vi "Init Events.vi"(8 "error in (no error)":errorcluster, 11 "BluelinesRedlines in":refnum<class "BluelinesRedlines.lvclass">) -> (0 "error out":errorcluster, 3 "BluelinesRedlines out":refnum<class "BluelinesRedlines.lvclass">)   [LabVIEW 2020, in "VolatusGUIElements.lvlib" / "BluelinesRedlines.lvclass"]
uses:
  BluelinesRedlines.lvclass
  Value Change Data.ctl
  BLRL Control.ctl
  Events.ctl
  BluelinesRedlines.lvclass/BluelinesRedlines.ctl
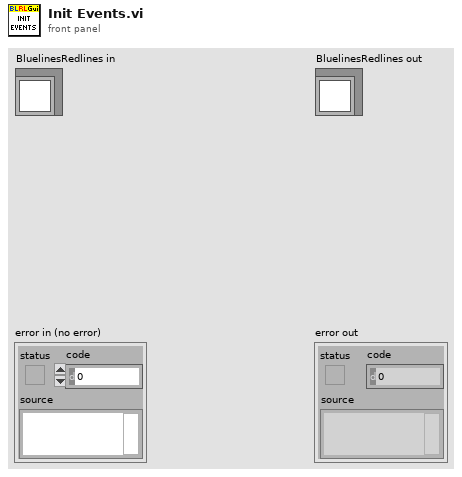
[diagram p1: front panel]
types:
  T1 = typedef "VolatusGUIElements.lvlib/BluelinesRedlines.lvclass/Events.ctl" = cluster{"Value Change":refnum<user-event>, "Disabled":refnum<user-event>}
  T2 = typedef "VolatusGUIElements.lvlib/BluelinesRedlines.lvclass/Value Change Data.ctl" = cluster{"Old":T3, "New":T3}
  T3 = typedef "VolatusGUIElements.lvlib/BluelinesRedlines.lvclass/BLRL Control.ctl" = cluster{"Blue Lines":cluster{"Channel":string, "Low":string, "Value":dbl, "High":string, "Color":u32, "Remove Channel":bool}[], "Red Lines":cluster{"Channel":string, "Low":string, "Value":dbl, "High":string, "Color":u32, "Remove Channel":bool}[], "Import":bool, "Export":bool, "Blueline Status":bool, "Redlines Status":bool, "Group":string, "New Group":bool, "Dup Group":bool, "Remove Group":bool, "Add Blue Channel":bool, "Add Red Channel":bool, "Reset Redlines":bool}
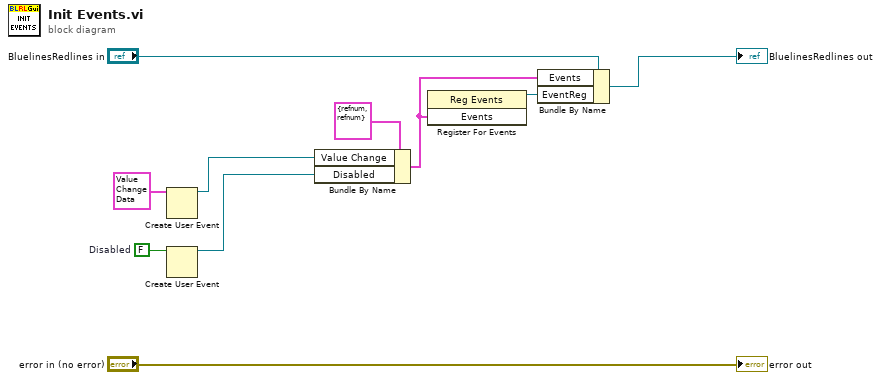
[diagram p0: block diagram]
diagram:
  w2 = FALSE  # Disabled
  n1 = Create User Event(user event datatype=T2 {"Old"={"Blue Lines"=[], "Red Lines"=[], "Import"=FALSE, "Export"=FALSE, "Blueline Status"=FALSE, "Redlines Status"=FALSE, "Group"="", "New Group"=FALSE, "Dup Group"=FALSE, "Remove Group"=FALSE, "Add Blue Channel"=FALSE, "Add Red Channel"=FALSE, "Reset Redlines"=FALSE}, "New"={"Blue Lines"=[], "Red Lines"=[], "Import"=FALSE, "Export"=FALSE, "Blueline Status"=FALSE, "Redlines Status"=FALSE, "Group"="", "New Group"=FALSE, "Dup Group"=FALSE, "Remove Group"=FALSE, "Add Blue Channel"=FALSE, "Add Red Channel"=FALSE, "Reset Redlines"=FALSE}} ("Value Change Data")) -> (user event=w6:refnum<user-event>)  [unwired: 1 in, 1 out]
  n2 = Create User Event(user event datatype=w2) -> (user event=w1:refnum<user-event>)  [unwired: 1 in, 1 out]
  n3 = Bundle By Name(cluster=T1 {"Value Change"=refnum, "Disabled"=refnum} ("Events"), "Value Change"=w6, "Disabled"=w1) -> (w4:T1)
  n4 = register-events(w4) -> (reference out=w3:refnum<event-registration>)  [unwired: 2 in, 1 out]
  n5 = Bundle By Name(cluster="BluelinesRedlines in", "Events"=w4, "EventReg"=w3) -> (→"BluelinesRedlines out":refnum<class "BluelinesRedlines.lvclass">)
  "error out" <- "error in (no error)"
